vi "Append To Log.vi"(8 "error in (no error)":errorcluster, 10 "String":string, 11 "Cooler Alternate UI in":refnum<class "Programmatic Controller.lvclass">) -> (0 "error out":errorcluster)   [LabVIEW 2025, in "Programmatic Controller.lvclass"]
doc: "Given a message, append to the ongoing log file. The caller is responsible for adding end of line characters to the text as desired."
uses:
  Programmatic Controller.lvclass
  Programmatic Controller.lvclass/Programmatic Controller.ctl
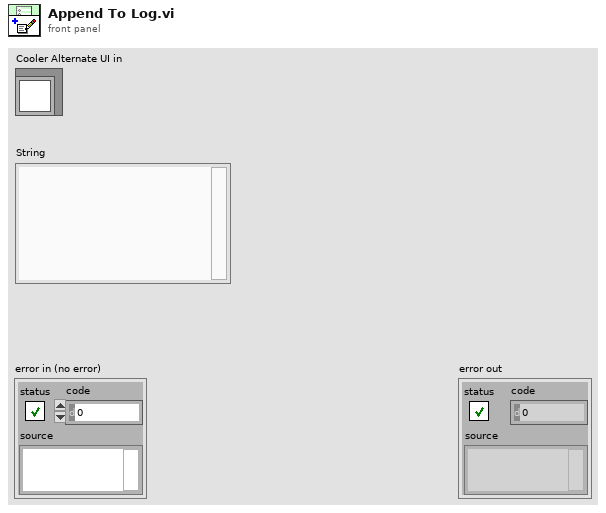
[diagram p1: front panel]
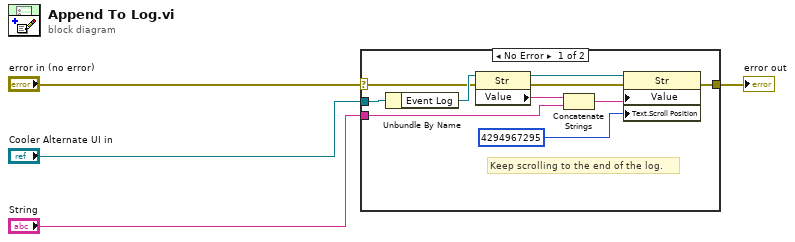
[diagram p0: block diagram]
diagram:
  n1 = case shown="No Error" "error in (no error)" {
    selector: "error in (no error)" -> [w10 w15]
    tunnel: [w9 w15] -> w3
    tunnel: "Cooler Alternate UI in" -> [w14 _]
    tunnel: "String" -> [w7 _]
    frame No Error {
      # "Keep scrolling to the end of the log."
      n2 = Unbundle By Name(w14) -> ("Event Log"=w13:refnum<vi>)
      n3 = property class="Str"(reference=w13, error in=w10) -> (reference out=w11:refnum<vi>, error out=w12:errorcluster, "Value"=w8:string)
      n4 = Concatenate Strings(w8, w7) -> (w6:string)
      n5 = property class="Str"(reference=w11, error in=w12, "Value"=w6, "Text.Scroll Position"=u32 4294967295) -> (error out=w9:errorcluster)  [unwired: 1 out]
    }
    frame Error {
    }
  }
  "error out" <- w3
